vi "pause (global variable).vi"() -> ()   [LabVIEW 2020, in "core.lvlib"]
uses:
  core.lvlib
panel:
  out "pause core?":bool
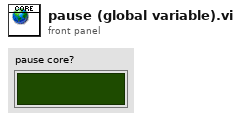
[diagram p1: front panel]
diagram:
